vi "Quad Encoder FPGA 7841.vi"() -> ()   [LabVIEW 8.6]
doc: "This VI contains a feature rich quadrature decoder with index support. The A, B, and Z values for the index state can be programmatically set, as well as counting direction for A and B. The current counter value is saved on every index state, and the counter is then reloaded. The counter can also be reset asynchronously with the reset button."
uses:
  <vilib>/Platform/TimedLoop/XDataNode/XDataNode.xnode
  <vilib>/Platform/TimedLoop/XDataNode/nitl_modes.ctl
  <vilib>/Platform/TimedLoop/XDataNode/XDNodeRunTimeDep.lvlib
  <vilib>/Platform/TimedLoop/XDataNode/wakeup.ctl
  <vilib>/Platform/TimedLoop/XDataNode/timing_clust.ctl
  <vilib>/eio/EIONode/EIONode.xnode
panel:
  out "Connector 1 DIO Port 0":u8
  out "Connector 1 DIO Port 1":u8
  out "Connector 1 DIO Port 2":u8
  out "Connector 1 DIO Port 3":u8
  out "Connector 1 DIO Port 4":u8
  in  "Connector 2 DIO Port 0":u8
  in  "Connector 2 DIO Port 1":u8
  in  "Connector 2 DIO Port 2":u8
  in  "Connector 2 DIO Port 3":u8
  in  "Connector 2 DIO Port 4":u8
  in  "stop":bool
  out "Encoder Position - Quad 7":i32
  in  "Reset - Quad 7":bool
  in  "Direction - Quad 7":bool
  in  "Period (Ticks) - Quad 7":u32
  out "Current Period - Quad 7":u32
  out "Period Count - Quad 7":u32
  in  "Input - Quad 7":bool
  out "Encoder Position - Quad 6":i32
  in  "Reset - Quad 6":bool
  in  "Direction - Quad 6":bool
  in  "Period (Ticks) - Quad 6":u32
  out "Current Period - Quad 6":u32
  out "Period Count - Quad 6":u32
  in  "Input - Quad 6":bool
  out "Encoder Position - Quad 5":i32
  in  "Reset - Quad 5":bool
  in  "Direction - Quad 5":bool
  in  "Period (Ticks) - Quad 5":u32
  out "Current Period - Quad 5":u32
  out "Period Count - Quad 5":u32
  in  "Input - Quad 5":bool
  out "Encoder Position - Quad 4":i32
  in  "Reset - Quad 4":bool
  in  "Direction - Quad 4":bool
  in  "Period (Ticks) - Quad 4":u32
  out "Current Period - Quad 4":u32
  out "Period Count - Quad 4":u32
  in  "Input - Quad 4":bool
  out "Encoder Position - Quad 3":i32
  in  "Reset - Quad 3":bool
  in  "Direction - Quad 3":bool
  in  "Period (Ticks) - Quad 3":u32
  out "Current Period - Quad 3":u32
  out "Period Count - Quad 3":u32
  in  "Input - Quad 3":bool
  out "Encoder Position - Quad 2":i32
  in  "Reset - Quad 2":bool
  in  "Direction - Quad 2":bool
  in  "Period (Ticks) - Quad 2":u32
  out "Current Period - Quad 2":u32
  out "Period Count - Quad 2":u32
  in  "Input - Quad 2":bool
  out "Encoder Position - Quad 1":i32
  in  "Reset - Quad 1":bool
  in  "Direction - Quad 1":bool
  in  "Period (Ticks) - Quad 1":u32
  out "Current Period - Quad 1":u32
  out "Period Count - Quad 1":u32
  in  "Input - Quad 1":bool
  in  "Input - Quad 0":bool
  out "Period Count - Quad 0":u32
  out "Current Period - Quad 0":u32
  in  "Period (Ticks) - Quad 0":u32
  in  "Direction - Quad 0":bool
  out "Encoder Position - Quad 0":i32
  in  "Reset - Quad 0":bool
  # "Quadrature Output"
  # "Quadrature Input"
  # "Quadrature Output"
  # "Quadrature Input"
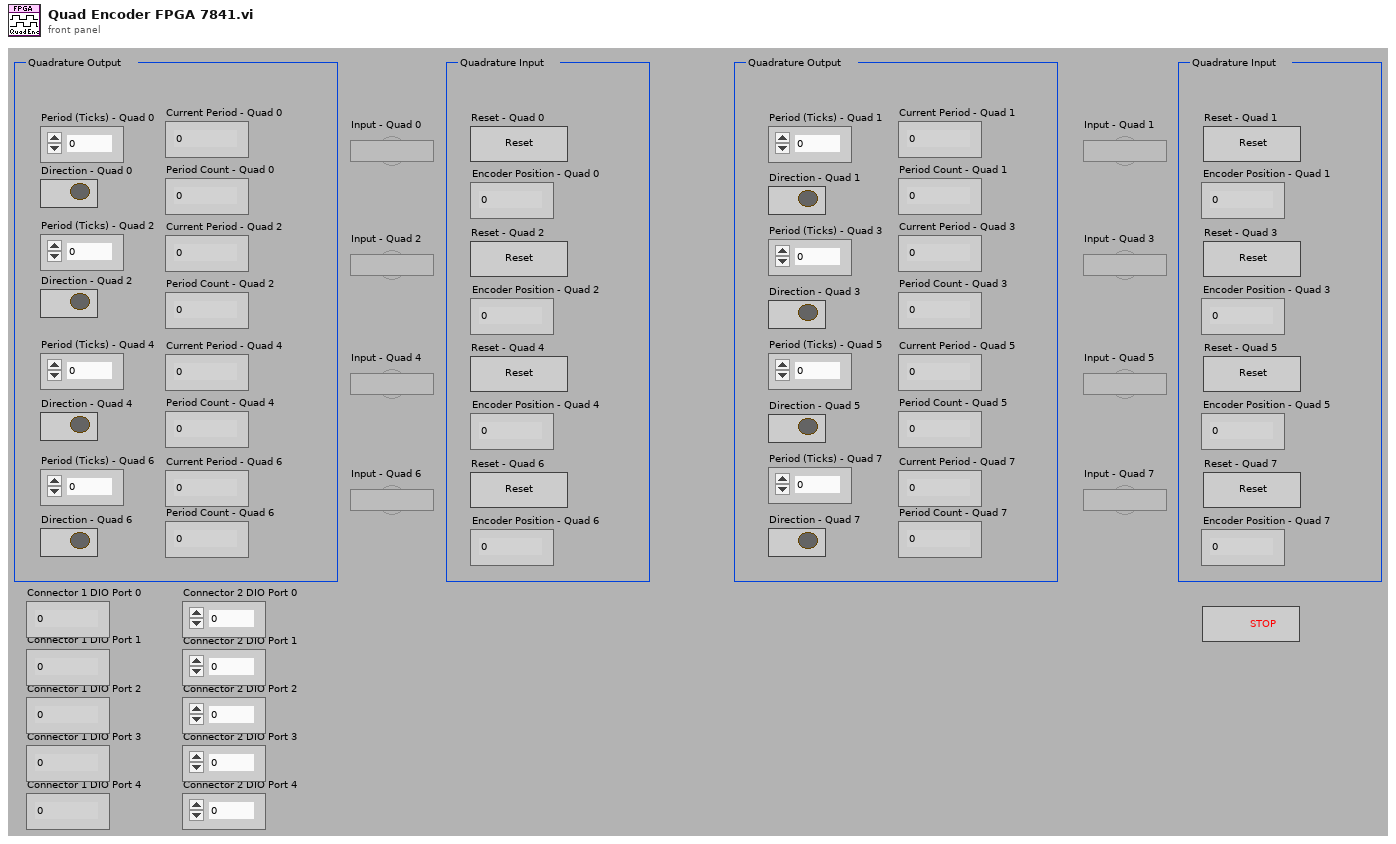
[diagram p1: front panel]
types:
  T1 = typedef "XDNodeRunTimeDep.lvlib/timing_clust.ctl" = cluster{"Expected End [f-1]":u64, "Actual End [f-1]":u64, "Finished Late? [f-1]":bool, "Expected End [i-1]":u64, "Actual End [i-1]":u64, "Finished Late? [i-1]":bool, "Expected Start [i]":u64, "Actual Start [i]":u64, "Expected Start [f]":u64, "Actual Start [f]":u64, "Source Name":string, "Structure Name":string, "Period":i64, "Deadline":i64, "Offset":i64, "Start":i64, "Priority":i32, "Timeout":i32, "Mode":T2, "Wakeup Reason":T3, "Error":errorcluster, "Source Type":string, "Secondary Source Type":string, "Global End Time":u64, "Global Start Time":u64, "Frame Duration":u64, "Iteration Duration":u64, "Assigned CPU":i32, "I/O Scan Engine Mode":u32}
  T2 = typedef "XDNodeRunTimeDep.lvlib/nitl_modes.ctl" = enum32{"No Change", "Process missed periods, maintain original phase", "Discard missed periods, maintain original phase", "Process missed periods, ignore original phase", "Discard missed periods, ignore original phase"}
  T3 = typedef "XDNodeRunTimeDep.lvlib/wakeup.ctl" = enum32{"Normal", "Aborted", "Asynchronous wakeup", "Timing source error", "Timed loop error", "Timeout"}
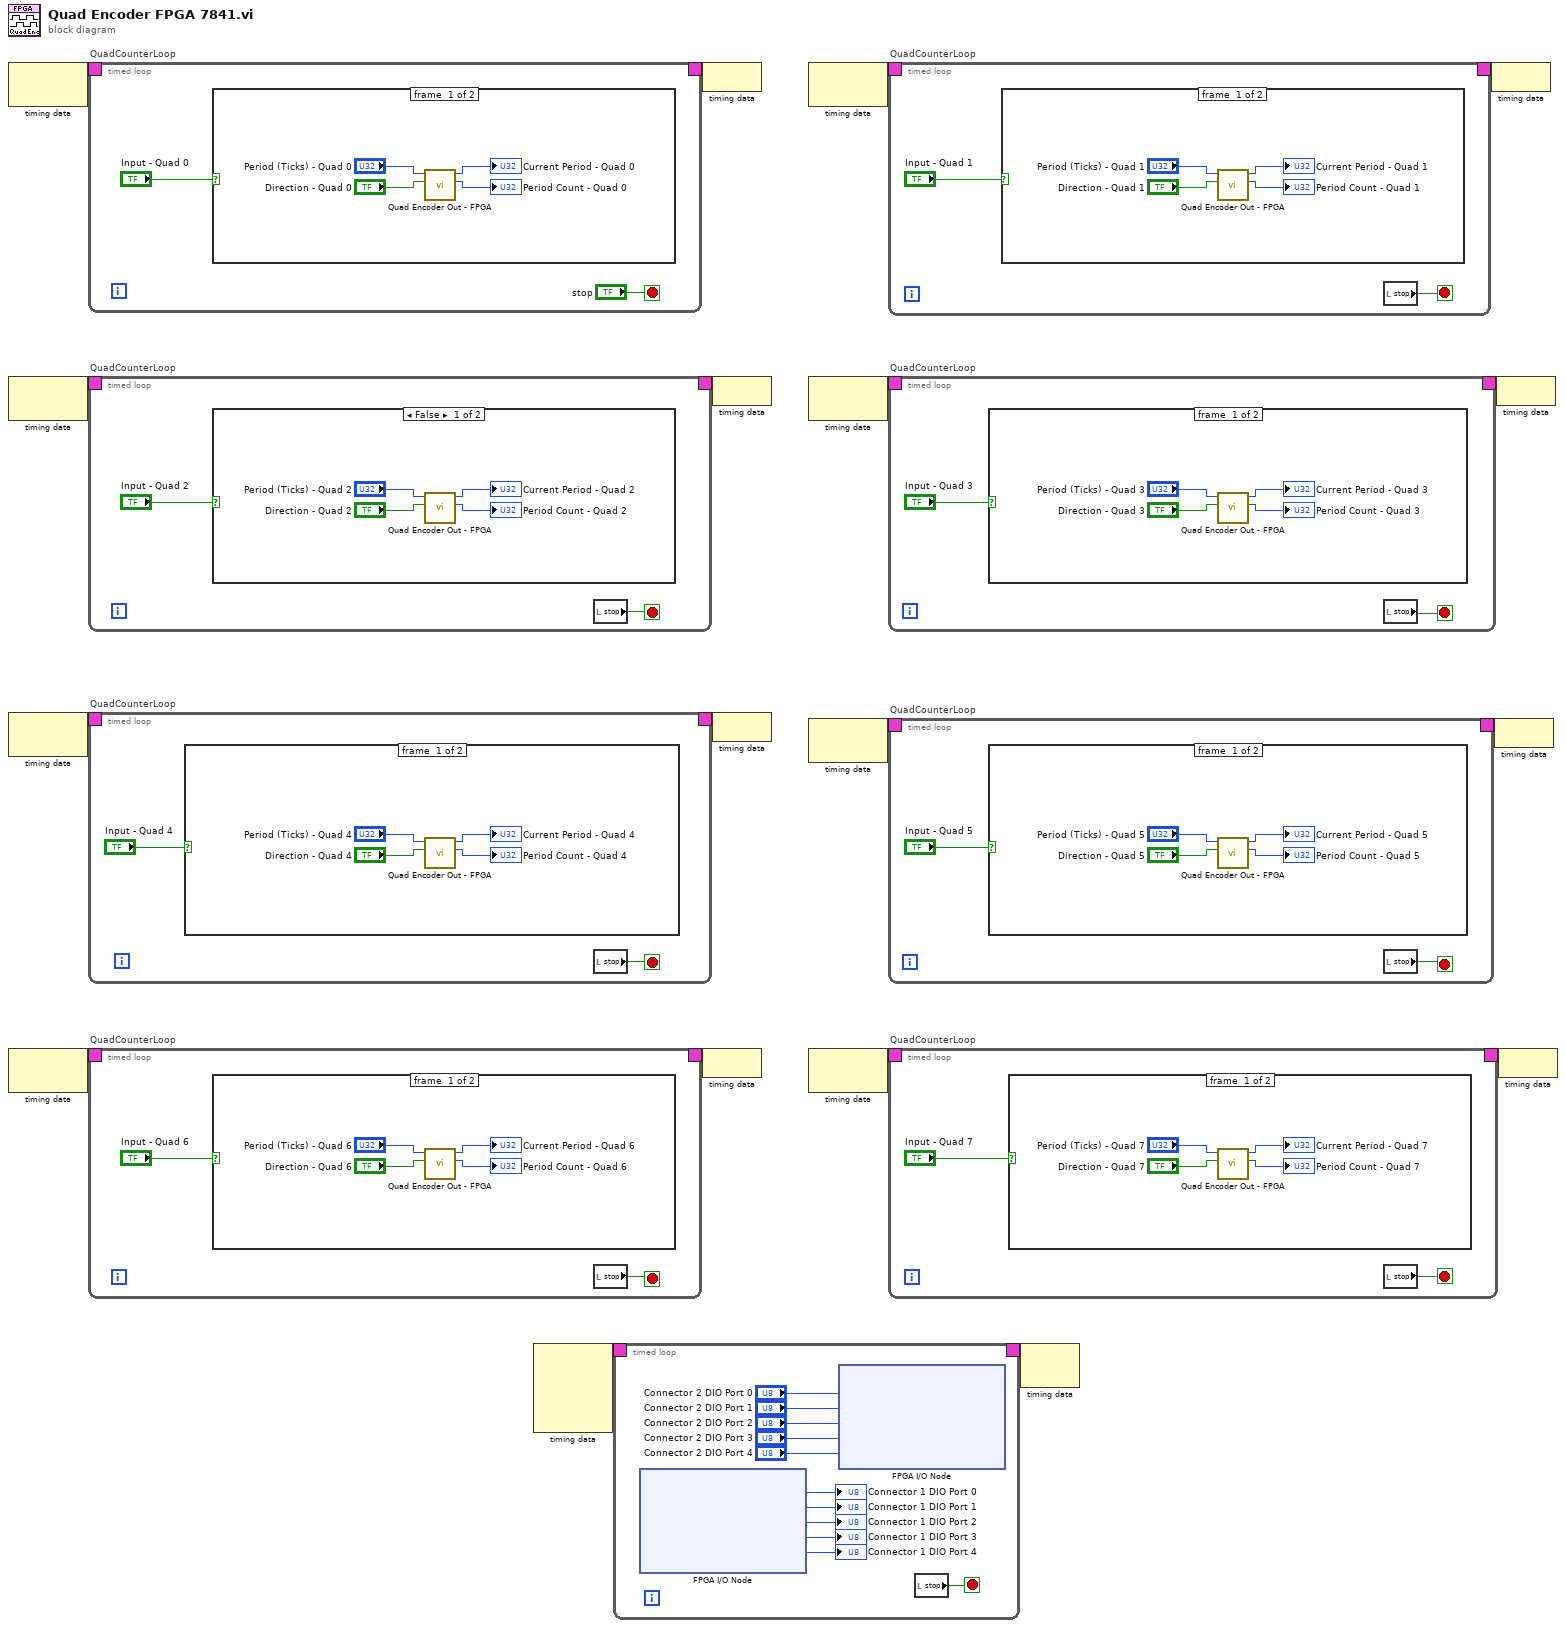
[diagram p0: block diagram]
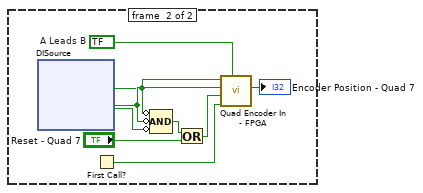
[diagram p2: hidden frame]
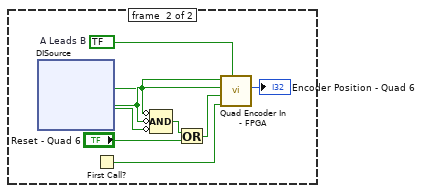
[diagram p3: hidden frame]
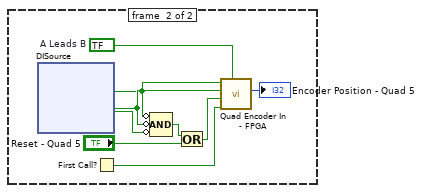
[diagram p4: hidden frame]
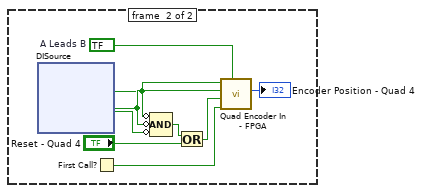
[diagram p5: hidden frame]
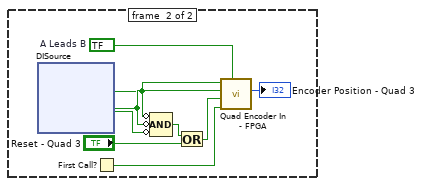
[diagram p6: hidden frame]
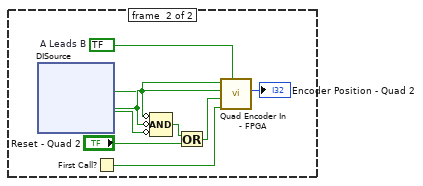
[diagram p7: hidden frame]
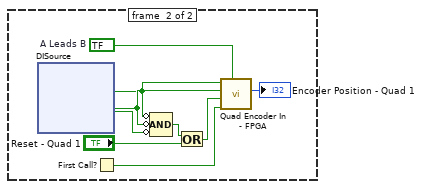
[diagram p8: hidden frame]
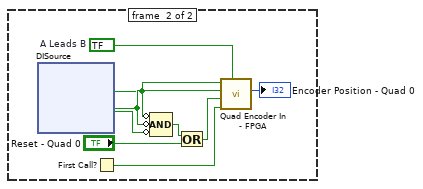
[diagram p9: hidden frame]
diagram:
  n1 = node-c288 ("Input Node")() -> (w18:T1)  [unwired: 1 in]
  n2 = node-c288 ("Input Node")() -> (w14:T1)  [unwired: 1 in]
  n3 = node-c288 ("Input Node")() -> (w10:T1)  [unwired: 1 in]
  n4 = node-c288 ("Input Node")() -> (w6:T1)  [unwired: 1 in]
  n5 = timed-loop "QuadCounterLoop" {
    timing-out: [_] -> w17
    timing: w18 -> [_]
    stop <- "stop" stop-if-true
    n6 = case shown="True" "Input - Quad 0" {
      frame #0 {
        n7 = call "Quad Encoder Out - FPGA.vi"("Direction ?"="Direction - Quad 0", "Period"="Period (Ticks) - Quad 0") -> ("Period Count"=→"Period Count - Quad 0":u32, "Current Period"=→"Current Period - Quad 0":u32)  [unwired: 8 in]
      }
      frame #1 {
        w25 = bool ?  # A Leads B
        n8 = xnode ("DISource")() -> ("DIO0"=w26:bool, "DIO1"=w27:bool, "DIO2"=w28:bool)  [unwired: 3 in, 3 out]
        n9 = First Call?() -> (First Call?: T/F=w33:bool)
        n10 = Compound Arithmetic op=AND(invert w26, invert w27, invert w28) -> (w29:bool)
        n11 = Or(x=w29, y="Reset - Quad 0") -> (x .or. y?=w32:bool)
        n12 = call "Quad Encoder In - FPGA.vi"("Direction?"=w25, "First Run?"=w33, "Reset"=w32, "Source B"=w27, "Source A"=w26) -> ("Position"=→"Encoder Position - Quad 0":i32)  [unwired: 6 in]
      }
    }
  }
  n13 = timed-loop "QuadCounterLoop" {
    timing-out: [_] -> w13
    timing: w14 -> [_]
    stop <- w36 stop-if-true
    n14 = case shown="False" "Input - Quad 2" {
      frame #0 {
        n15 = call "Quad Encoder Out - FPGA.vi"("Direction ?"="Direction - Quad 2", "Period"="Period (Ticks) - Quad 2") -> ("Period Count"=→"Period Count - Quad 2":u32, "Current Period"=→"Current Period - Quad 2":u32)  [unwired: 8 in]
      }
      frame #1 {
        w42 = bool ?  # A Leads B
        n16 = xnode ("DISource")() -> ("DIO0"=w43:bool, "DIO1"=w44:bool, "DIO2"=w45:bool)  [unwired: 3 in, 3 out]
        n17 = First Call?() -> (First Call?: T/F=w50:bool)
        n18 = Compound Arithmetic op=AND(invert w43, invert w44, invert w45) -> (w46:bool)
        n19 = Or(x=w46, y="Reset - Quad 2") -> (x .or. y?=w49:bool)
        n20 = call "Quad Encoder In - FPGA.vi"("Direction?"=w42, "First Run?"=w50, "Reset"=w49, "Source B"=w44, "Source A"=w43) -> ("Position"=→"Encoder Position - Quad 2":i32)  [unwired: 6 in]
      }
    }
    n21 = local read "stop"() -> (w36:bool)
  }
  n22 = timed-loop "QuadCounterLoop" {
    timing-out: [_] -> w9
    timing: w10 -> [_]
    stop <- w53 stop-if-true
    n23 = case shown="True" "Input - Quad 4" {
      frame #0 {
        n24 = call "Quad Encoder Out - FPGA.vi"("Direction ?"="Direction - Quad 4", "Period"="Period (Ticks) - Quad 4") -> ("Period Count"=→"Period Count - Quad 4":u32, "Current Period"=→"Current Period - Quad 4":u32)  [unwired: 8 in]
      }
      frame #1 {
        w59 = bool ?  # A Leads B
        n25 = xnode ("DISource")() -> ("DIO0"=w60:bool, "DIO1"=w61:bool, "DIO2"=w62:bool)  [unwired: 3 in, 3 out]
        n26 = First Call?() -> (First Call?: T/F=w67:bool)
        n27 = Compound Arithmetic op=AND(invert w60, invert w61, invert w62) -> (w63:bool)
        n28 = Or(x=w63, y="Reset - Quad 4") -> (x .or. y?=w66:bool)
        n29 = call "Quad Encoder In - FPGA.vi"("Direction?"=w59, "First Run?"=w67, "Reset"=w66, "Source B"=w61, "Source A"=w60) -> ("Position"=→"Encoder Position - Quad 4":i32)  [unwired: 6 in]
      }
    }
    n30 = local read "stop"() -> (w53:bool)
  }
  n31 = timed-loop "QuadCounterLoop" {
    timing-out: [_] -> w5
    timing: w6 -> [_]
    stop <- w70 stop-if-true
    n32 = case shown="True" "Input - Quad 6" {
      frame #0 {
        n33 = call "Quad Encoder Out - FPGA.vi"("Direction ?"="Direction - Quad 6", "Period"="Period (Ticks) - Quad 6") -> ("Period Count"=→"Period Count - Quad 6":u32, "Current Period"=→"Current Period - Quad 6":u32)  [unwired: 8 in]
      }
      frame #1 {
        w76 = bool ?  # A Leads B
        n34 = xnode ("DISource")() -> ("DIO0"=w77:bool, "DIO1"=w78:bool, "DIO2"=w79:bool)  [unwired: 3 in, 3 out]
        n35 = First Call?() -> (First Call?: T/F=w84:bool)
        n36 = Compound Arithmetic op=AND(invert w77, invert w78, invert w79) -> (w80:bool)
        n37 = Or(x=w80, y="Reset - Quad 6") -> (x .or. y?=w83:bool)
        n38 = call "Quad Encoder In - FPGA.vi"("Direction?"=w76, "First Run?"=w84, "Reset"=w83, "Source B"=w78, "Source A"=w77) -> ("Position"=→"Encoder Position - Quad 6":i32)  [unwired: 6 in]
      }
    }
    n39 = local read "stop"() -> (w70:bool)
  }
  n40 = node-c288() -> (w2:T1)  [unwired: 4 in]
  n41 = timed-loop "DIO Loop" {
    timing: w2 -> [_]
    timing-out: [_] -> w1
    stop <- w97 stop-if-true
    n42 = xnode "FPGA I/O Node"() -> ("Connector1/DIOPORT0"=→"Connector 1 DIO Port 0":u8, "Connector1/DIOPORT1"=→"Connector 1 DIO Port 1":u8, "Connector1/DIOPORT2"=→"Connector 1 DIO Port 2":u8, "Connector1/DIOPORT3"=→"Connector 1 DIO Port 3":u8, "Connector1/DIOPORT4"=→"Connector 1 DIO Port 4":u8)  [unwired: 5 in, 5 out]
    n43 = xnode "FPGA I/O Node"("Connector2/DIOPORT0"="Connector 2 DIO Port 0", "Connector2/DIOPORT1"="Connector 2 DIO Port 1", "Connector2/DIOPORT2"="Connector 2 DIO Port 2", "Connector2/DIOPORT3"="Connector 2 DIO Port 3", "Connector2/DIOPORT4"="Connector 2 DIO Port 4") -> ()  [unwired: 5 in, 5 out]
    n44 = local read "stop"() -> (w97:bool)
  }
  n45 = node-c288 ("Output Node")(w17) -> ()
  n46 = node-c288 ("Output Node")(w5) -> ()
  n47 = node-c288 ("Output Node")(w13) -> ()
  n48 = node-c288 ("Output Node")(w9) -> ()
  n49 = node-c288 ("Input Node")() -> (w16:T1)  [unwired: 1 in]
  n50 = node-c288 ("Input Node")() -> (w12:T1)  [unwired: 1 in]
  n51 = node-c288 ("Input Node")() -> (w8:T1)  [unwired: 1 in]
  n52 = node-c288 ("Input Node")() -> (w4:T1)  [unwired: 1 in]
  n53 = timed-loop "QuadCounterLoop" {
    timing-out: [_] -> w15
    timing: w16 -> [_]
    stop <- w100 stop-if-true
    n54 = case shown="True" "Input - Quad 1" {
      frame #0 {
        n55 = call "Quad Encoder Out - FPGA.vi"("Direction ?"="Direction - Quad 1", "Period"="Period (Ticks) - Quad 1") -> ("Period Count"=→"Period Count - Quad 1":u32, "Current Period"=→"Current Period - Quad 1":u32)  [unwired: 8 in]
      }
      frame #1 {
        w106 = bool ?  # A Leads B
        n56 = xnode ("DISource")() -> ("DIO0"=w107:bool, "DIO1"=w108:bool, "DIO2"=w109:bool)  [unwired: 3 in, 3 out]
        n57 = First Call?() -> (First Call?: T/F=w114:bool)
        n58 = Compound Arithmetic op=AND(invert w107, invert w108, invert w109) -> (w110:bool)
        n59 = Or(x=w110, y="Reset - Quad 1") -> (x .or. y?=w113:bool)
        n60 = call "Quad Encoder In - FPGA.vi"("Direction?"=w106, "First Run?"=w114, "Reset"=w113, "Source B"=w108, "Source A"=w107) -> ("Position"=→"Encoder Position - Quad 1":i32)  [unwired: 6 in]
      }
    }
    n61 = local read "stop"() -> (w100:bool)
  }
  n62 = timed-loop "QuadCounterLoop" {
    timing-out: [_] -> w11
    timing: w12 -> [_]
    stop <- w117 stop-if-true
    n63 = case shown="True" "Input - Quad 3" {
      frame #0 {
        n64 = call "Quad Encoder Out - FPGA.vi"("Direction ?"="Direction - Quad 3", "Period"="Period (Ticks) - Quad 3") -> ("Period Count"=→"Period Count - Quad 3":u32, "Current Period"=→"Current Period - Quad 3":u32)  [unwired: 8 in]
      }
      frame #1 {
        w123 = bool ?  # A Leads B
        n65 = xnode ("DISource")() -> ("DIO0"=w124:bool, "DIO1"=w125:bool, "DIO2"=w126:bool)  [unwired: 3 in, 3 out]
        n66 = First Call?() -> (First Call?: T/F=w131:bool)
        n67 = Compound Arithmetic op=AND(invert w124, invert w125, invert w126) -> (w127:bool)
        n68 = Or(x=w127, y="Reset - Quad 3") -> (x .or. y?=w130:bool)
        n69 = call "Quad Encoder In - FPGA.vi"("Direction?"=w123, "First Run?"=w131, "Reset"=w130, "Source B"=w125, "Source A"=w124) -> ("Position"=→"Encoder Position - Quad 3":i32)  [unwired: 6 in]
      }
    }
    n70 = local read "stop"() -> (w117:bool)
  }
  n71 = timed-loop "QuadCounterLoop" {
    timing-out: [_] -> w7
    timing: w8 -> [_]
    stop <- w134 stop-if-true
    n72 = case shown="True" "Input - Quad 5" {
      frame #0 {
        n73 = call "Quad Encoder Out - FPGA.vi"("Direction ?"="Direction - Quad 5", "Period"="Period (Ticks) - Quad 5") -> ("Period Count"=→"Period Count - Quad 5":u32, "Current Period"=→"Current Period - Quad 5":u32)  [unwired: 8 in]
      }
      frame #1 {
        w140 = bool ?  # A Leads B
        n74 = xnode ("DISource")() -> ("DIO0"=w141:bool, "DIO1"=w142:bool, "DIO2"=w143:bool)  [unwired: 3 in, 3 out]
        n75 = First Call?() -> (First Call?: T/F=w148:bool)
        n76 = Compound Arithmetic op=AND(invert w141, invert w142, invert w143) -> (w144:bool)
        n77 = Or(x=w144, y="Reset - Quad 5") -> (x .or. y?=w147:bool)
        n78 = call "Quad Encoder In - FPGA.vi"("Direction?"=w140, "First Run?"=w148, "Reset"=w147, "Source B"=w142, "Source A"=w141) -> ("Position"=→"Encoder Position - Quad 5":i32)  [unwired: 6 in]
      }
    }
    n79 = local read "stop"() -> (w134:bool)
  }
  n80 = timed-loop "QuadCounterLoop" {
    timing-out: [_] -> w3
    timing: w4 -> [_]
    stop <- w151 stop-if-true
    n81 = case shown="True" "Input - Quad 7" {
      frame #0 {
        n82 = call "Quad Encoder Out - FPGA.vi"("Direction ?"="Direction - Quad 7", "Period"="Period (Ticks) - Quad 7") -> ("Period Count"=→"Period Count - Quad 7":u32, "Current Period"=→"Current Period - Quad 7":u32)  [unwired: 8 in]
      }
      frame #1 {
        w157 = bool ?  # A Leads B
        n83 = xnode ("DISource")() -> ("DIO0"=w158:bool, "DIO1"=w159:bool, "DIO2"=w160:bool)  [unwired: 3 in, 3 out]
        n84 = First Call?() -> (First Call?: T/F=w165:bool)
        n85 = Compound Arithmetic op=AND(invert w158, invert w159, invert w160) -> (w161:bool)
        n86 = Or(x=w161, y="Reset - Quad 7") -> (x .or. y?=w164:bool)
        n87 = call "Quad Encoder In - FPGA.vi"("Direction?"=w157, "First Run?"=w165, "Reset"=w164, "Source B"=w159, "Source A"=w158) -> ("Position"=→"Encoder Position - Quad 7":i32)  [unwired: 6 in]
      }
    }
    n88 = local read "stop"() -> (w151:bool)
  }
  n89 = node-c288(w1) -> ()  [unwired: 1 out]
  n90 = node-c288 ("Output Node")(w15) -> ()
  n91 = node-c288 ("Output Node")(w7) -> ()
  n92 = node-c288 ("Output Node")(w11) -> ()
  n93 = node-c288 ("Output Node")(w3) -> ()
